vi "CRYPEAQ GL.vi"(8 "Lp":dbl=44100.0, 9 "fcN":dbl=1019.5, 10 "Amax":dbl=32768.0, 11 "NF":dbl=92.0) -> (3 "GL":dbl)   [LabVIEW 2013]
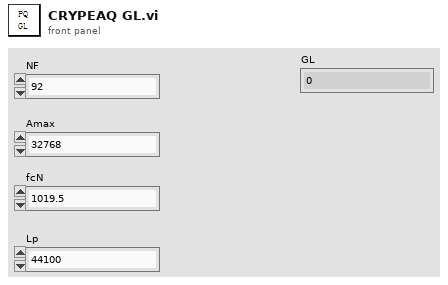
[diagram p1: front panel]
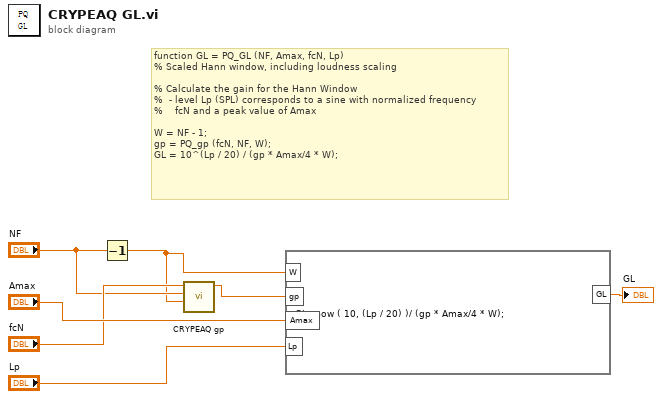
[diagram p0: block diagram]
diagram:
  # "function GL = PQ_GL (NF, Amax, fcN, Lp)\n% Scaled Hann window, including loudness scaling\n\n% Calculate the gain for the Hann Window\n%  - level Lp (SPL) corresponds to a sine with normalized frequency\n%    fcN and a peak value of Amax\n\nW = NF - 1;\ngp = PQ_gp (fcN, NF, W);\nGL = 10^(Lp / 20) / (gp * Amax/4 * W);"
  n1 = Decrement(x="NF") -> (x-1=w2:dbl)
  n2 = call "CRYPEAQ gp.vi"("W"=w2, "NF"="NF", "fcN"="fcN") -> ("gp"=w1:dbl)  [unwired: 8 in]
  n3 = formula code="GL=pow ( 10, (Lp / 20) )/ (gp * Amax/4 * W);"("Lp"="Lp", "gp"=w1, "Amax"="Amax", "W"=w2) -> ("GL"=→"GL":dbl)
